vi "KnowPosition.vi"() -> ()   [LabVIEW 2019]
uses:
  refnums.vi
  dsinstructions.vi
  sensors.vi
  dsdata.vi
  autoinfo.vi
panel:
  out "Y Position (in)":dbl
  out "X Position (in)":dbl
  out "Robot Position":cluster{dbl[], dbl[]}(graph)
  out "Heading (deg)":dbl format="%#_13g"
  in  "Plot Data":bool
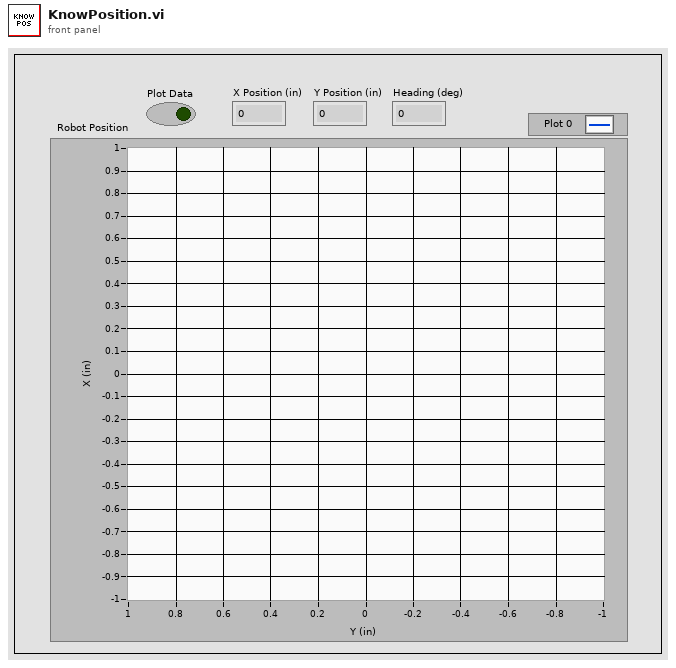
[diagram p1: front panel]
types:
  T1 = typedef "WPI_MotorControlDeviceRef.ctl" = cluster{"DeviceStatus":errorcluster, "Type":T2, "PWM":cluster{"PWM Channel":T3, "DeadBand":T4}, "CAN":cluster{"Device Number":u8, "SetOutput VI Ref":variant, "GetOutput VI Ref":variant, "Enable VI Ref":variant, "Disable VI Ref":variant, "Data":variant}, "Invert":bool, "DIO PWM":cluster{"PWM \"Enable\" Channel":T3, "DIOChannel":T5, "PWM Rate":dbl}}
  T2 = typedef "WPI_MotorControlType.ctl" = enum16{"PWM", "CAN", "DIO PWM"}
  T3 = typedef "FPGA_DIOPWMChannel.ctl" = enum8{"PWM 0", "PWM 1", "PWM 2", "PWM 3", "PWM 4", "PWM 5", "PWM 6", "PWM 7", "PWM 8", "PWM 9", "PWM MXP 0", "PWM MXP 1", "PWM MXP 2", "PWM MXP 3", "PWM MXP 4", "PWM MXP 5", "PWM MXP 6", "PWM MXP 7", "PWM MXP 8", "PWM MXP 9", "Invalid"}
  T4 = typedef "WPI_PWMDeadband.ctl" = cluster{"Name":string, "maxPositivePwm":i32, "minPositivePwm":i32, "centerPwm":i32, "maxNegativePwm":i32, "minNegativePwm":i32, "angularRange":u16}
  T5 = typedef "FPGA_DIOChannel.ctl" = enum8{"DIO 0", "DIO 1", "DIO 2", "DIO 3", "DIO 4", "DIO 5", "DIO 6", "DIO 7", "DIO 8", "DIO 9", "DIO MXP 0", "DIO MXP 1", "DIO MXP 2", "DIO MXP 3", "DIO MXP 4", "DIO MXP 5", "DIO MXP 6", "DIO MXP 7", "DIO MXP 8", "DIO MXP 9", "DIO MXP 10", "DIO MXP 11", "DIO MXP 12", "DIO MXP 13", "DIO MXP 14", "DIO MXP 15", "SPI Port CS1", "SPI Port CS2", "SPI Port CS3", "SPI Port MISO", "SPI Port MOSI", "Invalid"}
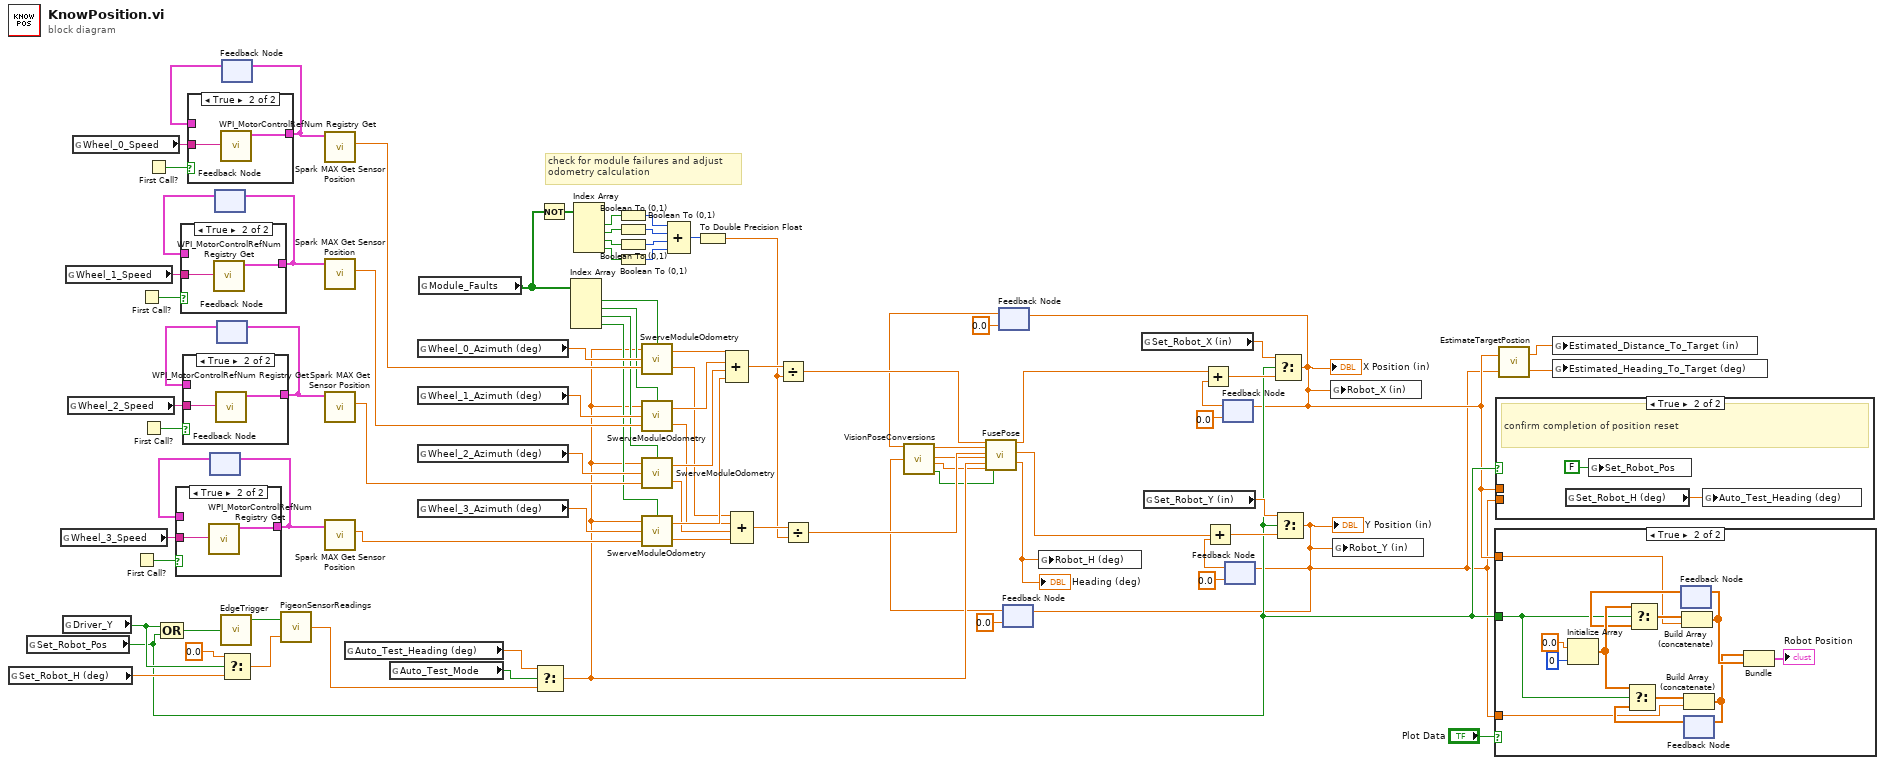
[diagram p0: block diagram]
diagram:
  # "check for module failures and adjust\nodometry calculation"
  n1 = global read "sensors.vi" "Set_Robot_H (deg)"() -> (w44:dbl)
  n2 = global read "sensors.vi" "Set_Robot_Pos"() -> (w19:bool)
  n3 = global read "refnums.vi" "Wheel_3_Speed"() -> (w76:string)
  n4 = global read "dsinstructions.vi" "Driver_Y"() -> (w43:bool)
  n5 = global read "refnums.vi" "Wheel_1_Speed"() -> (w82:string)
  n6 = global read "refnums.vi" "Wheel_2_Speed"() -> (w79:string)
  n7 = global read "refnums.vi" "Wheel_0_Speed"() -> (w85:string)
  n8 = First Call?() -> (First Call?: T/F=w78:bool)
  n9 = First Call?() -> (First Call?: T/F=w84:bool)
  n10 = First Call?() -> (First Call?: T/F=w81:bool)
  n11 = First Call?() -> (First Call?: T/F=w87:bool)
  n12 = Compound Arithmetic op=OR(w43, w19) -> (w42:bool)
  n13 = feedback #1() -> (w77:T1)  [unwired: 1 in]
  n14 = case shown="True" w78 {
    tunnel: [w88 w89] -> w73
    tunnel: w77 -> [w88 _]
    tunnel: w76 -> [_ w90]
    frame False {
    }
    frame True {
      n15 = call <vilib>:"WPI_MotorControlRefNum Registry Get.vi"("refnum name"=w90) -> ("MotorControlDevRef"=w89:T1)  [unwired: 9 in, 1 out]
    }
  }
  n16 = feedback-in #1(w73) -> ()
  n17 = feedback #2() -> (w83:T1)  [unwired: 1 in]
  n18 = case shown="True" w84 {
    tunnel: [w91 w92] -> w75
    tunnel: w83 -> [w91 _]
    tunnel: w82 -> [_ w93]
    frame False {
    }
    frame True {
      n19 = call <vilib>:"WPI_MotorControlRefNum Registry Get.vi"("refnum name"=w93) -> ("MotorControlDevRef"=w92:T1)  [unwired: 9 in, 1 out]
    }
  }
  n20 = feedback-in #2(w75) -> ()
  n21 = feedback #3() -> (w80:T1)  [unwired: 1 in]
  n22 = case shown="True" w81 {
    tunnel: [w94 w95] -> w74
    tunnel: w80 -> [w94 _]
    tunnel: w79 -> [_ w96]
    frame False {
    }
    frame True {
      n23 = call <vilib>:"WPI_MotorControlRefNum Registry Get.vi"("refnum name"=w96) -> ("MotorControlDevRef"=w95:T1)  [unwired: 9 in, 1 out]
    }
  }
  n24 = feedback-in #3(w74) -> ()
  n25 = call "EdgeTrigger.vi"("Input Signal"=w42) -> ("Rising Edge Trigger"=w41:bool)  [unwired: 2 out]
  n26 = feedback #4() -> (w86:T1)  [unwired: 1 in]
  n27 = case shown="True" w87 {
    tunnel: [w97 w98] -> w72
    tunnel: w86 -> [w97 _]
    tunnel: w85 -> [_ w99]
    frame False {
    }
    frame True {
      n28 = call <vilib>:"WPI_MotorControlRefNum Registry Get.vi"("refnum name"=w99) -> ("MotorControlDevRef"=w98:T1)  [unwired: 9 in, 1 out]
    }
  }
  n29 = feedback-in #4(w72) -> ()
  n30 = Select(t=0.0 ("f"), s=w43, f=w44) -> (s? t:f=w46:dbl)
  n31 = call "PigeonSensorReadings.vi"("Reset Yaw (deg)"=w46, "Reset Yaw"=w41) -> ("Yaw (deg)"=w22:dbl)
  n32 = call <vilib>:"Spark MAX Get Sensor Position.vi"("MotorControlDevRef in"=w72) -> ("Sensor Position"=w70:dbl)  [unwired: 7 in, 3 out]
  n33 = call <vilib>:"Spark MAX Get Sensor Position.vi"("MotorControlDevRef in"=w75) -> ("Sensor Position"=w68:dbl)  [unwired: 7 in, 3 out]
  n34 = call <vilib>:"Spark MAX Get Sensor Position.vi"("MotorControlDevRef in"=w74) -> ("Sensor Position"=w67:dbl)  [unwired: 7 in, 3 out]
  n35 = call <vilib>:"Spark MAX Get Sensor Position.vi"("MotorControlDevRef in"=w73) -> ("Sensor Position"=w39:dbl)  [unwired: 7 in, 3 out]
  n36 = global read "autoinfo.vi" "Auto_Test_Heading (deg)"() -> (w20:dbl)
  n37 = global read "dsdata.vi" "Auto_Test_Mode"() -> (w21:bool)
  n38 = global read "sensors.vi" "Wheel_0_Azimuth (deg)"() -> (w69:dbl)
  n39 = global read "sensors.vi" "Wheel_1_Azimuth (deg)"() -> (w66:dbl)
  n40 = global read "sensors.vi" "Wheel_2_Azimuth (deg)"() -> (w65:dbl)
  n41 = global read "sensors.vi" "Wheel_3_Azimuth (deg)"() -> (w40:dbl)
  n42 = global read "sensors.vi" "Module_Faults"() -> (w38:bool[])
  n43 = Select(t=w20, s=w21, f=w22) -> (s? t:f=w13:dbl)
  n44 = Not(x=w38) -> (.not. x?=w37:bool[])
  n45 = Index Array(array=w38) -> (element #1=w26:bool, element #2=w25:bool, element #3=w24:bool, element #4=w23:bool)  [unwired: 4 in]
  n46 = Index Array(array=w37) -> (element #1=w36:bool, element #2=w35:bool, element #3=w34:bool, element #4=w33:bool)  [unwired: 4 in]
  n47 = Boolean To (0,1)(Boolean=w36) -> (0, 1=w32:i16)
  n48 = Boolean To (0,1)(Boolean=w35) -> (0, 1=w31:i16)
  n49 = Boolean To (0,1)(Boolean=w34) -> (0, 1=w30:i16)
  n50 = Boolean To (0,1)(Boolean=w33) -> (0, 1=w29:i16)
  n51 = call "SwerveModuleOdometry.vi"("Module Fault"=w26, "Wheel Distance (native)"=w70, "Wheel Azimuth (deg)"=w69, "Robot Heading(deg)"=w13) -> ("Delta Y (in)"=w55:dbl, "Delta X (in)"=w64:dbl)
  n52 = call "SwerveModuleOdometry.vi"("Module Fault"=w25, "Wheel Distance (native)"=w68, "Wheel Azimuth (deg)"=w66, "Robot Heading(deg)"=w13) -> ("Delta Y (in)"=w56:dbl, "Delta X (in)"=w63:dbl)
  n53 = call "SwerveModuleOdometry.vi"("Module Fault"=w24, "Wheel Distance (native)"=w67, "Wheel Azimuth (deg)"=w65, "Robot Heading(deg)"=w13) -> ("Delta Y (in)"=w57:dbl, "Delta X (in)"=w62:dbl)
  n54 = call "SwerveModuleOdometry.vi"("Module Fault"=w23, "Wheel Distance (native)"=w39, "Wheel Azimuth (deg)"=w40, "Robot Heading(deg)"=w13) -> ("Delta Y (in)"=w58:dbl, "Delta X (in)"=w61:dbl)
  n55 = Compound Arithmetic op=ADD(w32, w31, w30, w29) -> (w28:i16)
  n56 = To Double Precision Float(number=w28) -> (double precision float=w27:dbl)
  n57 = Compound Arithmetic op=ADD(w64, w63, w62, w61) -> (w60:dbl)
  n58 = Compound Arithmetic op=ADD(w55, w56, w57, w58) -> (w59:dbl)
  n59 = Divide(x=w60, y=w27) -> (x/y=w18:dbl)
  n60 = Divide(x=w59, y=w27) -> (x/y=w14:dbl)
  n61 = feedback #5(0.0 ("Set_Robot_X (in)")) -> (w7:dbl)
  n62 = feedback #6(0.0 ("Set_Robot_Y (in)")) -> (w8:dbl)
  n63 = call "VisionPoseConversions.vi"("Current X Estimate (in)"=w7, "Current Y Estimate (in)"=w8) -> ("deltaX (in)"=w10:dbl, "deltaY (in)"=w11:dbl, "H (deg)"=w12:dbl, "Synced LimeLight Valid"=w5:bool)  [unwired: 1 in]
  n64 = call "FusePose.vi"("Odometry deltaX"=w18, "LimeLight deltaX"=w10, "Odometry deltaY"=w14, "LimeLight deltaY"=w11, "Odometry H"=w13, "LimeLight H"=w12, "LimeLight Valid"=w5) -> ("Fused deltaX"=w17:dbl, "Fused deltaY"=w16:dbl, "Fused H"=w15:dbl)  [unwired: 10 in]
  "Heading (deg)" <- w15
  n65 = global write "sensors.vi" "Robot_H (deg)"(w15) -> ()
  n66 = global read "sensors.vi" "Set_Robot_X (in)"() -> (w51:dbl)
  n67 = global read "sensors.vi" "Set_Robot_Y (in)"() -> (w47:dbl)
  n68 = feedback #7(0.0) -> (w54:dbl)
  n69 = Add(x=w17, y=w54) -> (x+y=w52:dbl)
  n70 = feedback #8(0.0) -> (w50:dbl)
  n71 = Add(x=w16, y=w50) -> (x+y=w48:dbl)
  n72 = Select(t=w51, s=w19, f=w52) -> (s? t:f=w4:dbl)
  "X Position (in)" <- w4
  n73 = feedback-in #5(w4) -> ()
  n74 = feedback-in #7(w4) -> ()
  n75 = Select(t=w47, s=w19, f=w48) -> (s? t:f=w3:dbl)
  "Y Position (in)" <- w3
  n76 = feedback-in #6(w3) -> ()
  n77 = feedback-in #8(w3) -> ()
  n78 = global write "sensors.vi" "Robot_X (in)"(w4) -> ()
  n79 = global write "sensors.vi" "Robot_Y (in)"(w3) -> ()
  n80 = case shown="True" "Plot Data" {
    tunnel: w19 -> [_ w100]
    tunnel: w4 -> [_ w103]
    tunnel: w3 -> [_ w102]
    frame False {
    }
    frame True {
      n81 = Initialize Array(0.0 ("element"), 0 ("dimension size")) -> (w112:dbl[])
      n82 = feedback #9() -> (w108:dbl[])  [unwired: 1 in]
      n83 = Select(t=w112, s=w100, f=w108) -> (s? t:f=w109:dbl[])
      n84 = Build Array (concatenate)(w109, w103) -> (w107:dbl[])
      n85 = feedback-in #9(w107) -> ()
      n86 = feedback #10() -> (w110:dbl[])  [unwired: 1 in]
      n87 = Select(t=w112, s=w100, f=w110) -> (s? t:f=w111:dbl[])
      n88 = Build Array (concatenate)(w111, w102) -> (w106:dbl[])
      n89 = feedback-in #10(w106) -> ()
      n90 = Bundle(w106, w107) -> (→"Robot Position":cluster{dbl[], dbl[]})  [unwired: 1 in]
    }
  }
  n91 = case shown="True" w19 {
    tunnel: w4 -> [_ _]
    tunnel: w3 -> [_ _]
    frame False {
    }
    frame True {
      # "confirm completion of position reset"
      n92 = global read "sensors.vi" "Set_Robot_H (deg)"() -> (w113:dbl)
      n93 = global write "sensors.vi" "Set_Robot_Pos"(FALSE ("Set_Robot_Pos")) -> ()
      n94 = global write "autoinfo.vi" "Auto_Test_Heading (deg)"(w113) -> ()
    }
  }
  n95 = call "EstimateTargetPostion.vi"("Robot Y (in)"=w3, "Robot X (in)"=w4) -> ("Estimated Heading to Target (deg)"=w1:dbl, "Estimated Distance to Target (in)"=w2:dbl)
  n96 = global write "sensors.vi" "Estimated_Distance_To_Target (in)"(w2) -> ()
  n97 = global write "sensors.vi" "Estimated_Heading_To_Target (deg)"(w1) -> ()
